vi "Workspace.Initialize.vi"(11 "State":T1) -> (0 "error out":errorcluster, 3 "State":T1)   [LabVIEW 2015, in "J1939 Workspace Object.lvlib"]
uses:
  J1939 Workspace Object.lvlib
  Control Addon/Source/Workspace Objects/Types/UI.StateVariables.ctl
  <vilib>/NI Veristand/Display Template Support/Display Template Support.llb/enum_Display Template Handler Minimal To Widget Msg.ctl
  <vilib>/NI Veristand/Execution/Workspace/SystemStateRegEventRef.ctl
  <vilib>/NI Veristand/Execution/Workspace/Target State Info.ctl
  <vilib>/NI Veristand/Execution/Workspace/Target State.ctl
  Shared/Types/Private Data.ctl
  <vilib>/NI/STM/TCP/TCP Connection Info.ctl
  <vilib>/NI/STM/SubVIs/MetaDataElement.ctl
  Shared/Types/Error Cluster.ctl
  Shared/Types/Error Types.ctl
  NationalInstruments.VeriStand.SystemStorage
  <vilib>/NI Veristand/Display Template Support/Display Template Support.llb/enum_Display Template Handler Minimal To Workspace.ctl
  <vilib>/NI Veristand/Execution/Workspace/WorkspaceAPI.ctl
  NationalInstruments.VeriStand.ClientAPI
  <vilib>/NI Veristand/Execution/Workspace/SystemStateEventRef.ctl
  Control Addon/Source/Workspace Objects/Types/UI.Refs.ctl
  <vilib>/NI Veristand/Execution/Workspace/NI_VS Workspace ExecutionAPI.lvlib
  Shared/J1939 Addon Shared.lvlib
  <vilib>/NI/STM/NI STM.lvlib
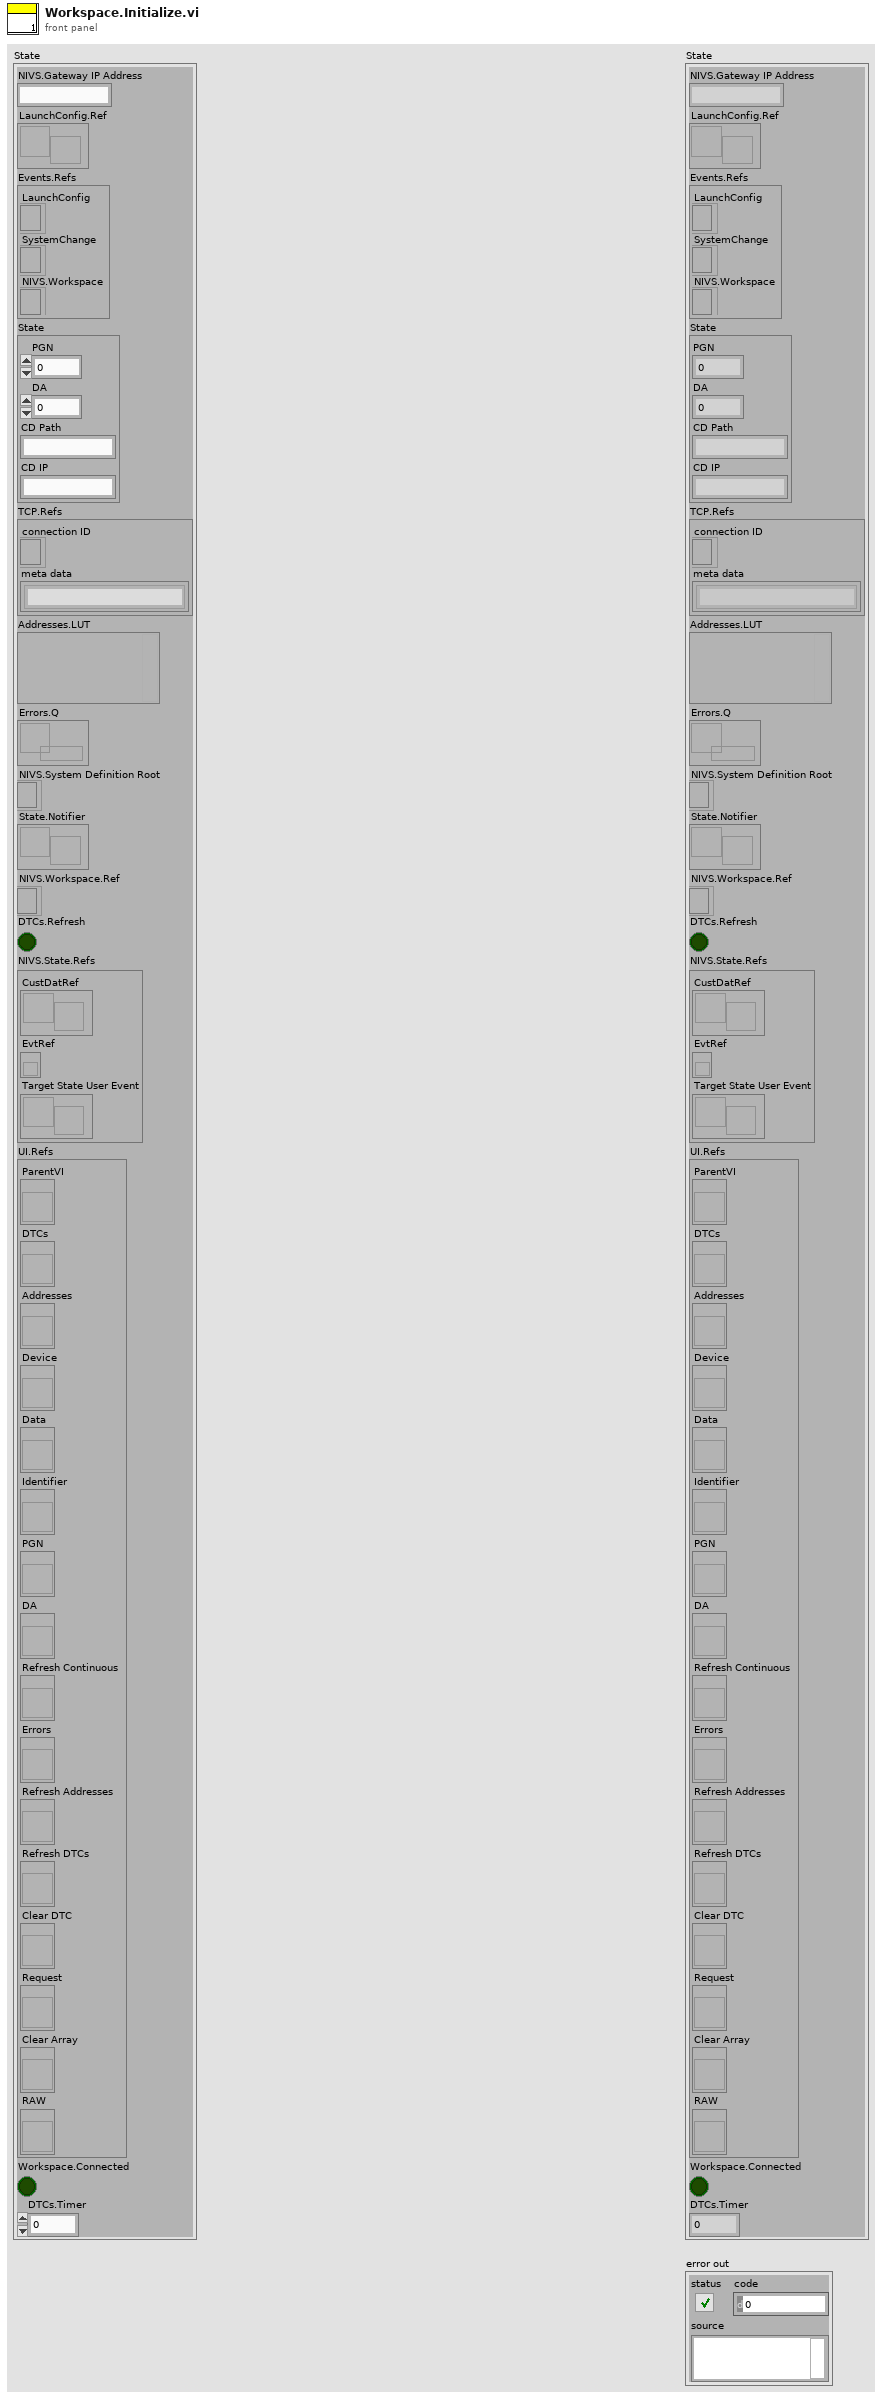
[diagram p1: front panel]
types:
  T1 = typedef "J1939 Workspace Object.lvlib/UI.StateVariables.ctl" = cluster{"NIVS.Gateway IP Address":string, "LaunchConfig.Ref":refnum<user-event>, "Events.Refs":cluster{"LaunchConfig":refnum<event-registration>, "SystemChange":T2, "NIVS.Workspace":refnum<event-registration>}, "State":T3, "TCP.Refs":T4, "Addresses.LUT":variant, "Errors.Q":refnum<queue>, "NIVS.System Definition Root":refnum<k24>, "State.Notifier":refnum<user-event>, "NIVS.Workspace.Ref":T6, "DTCs.Refresh":bool, "NIVS.State.Refs":T7, "UI.Refs":T8, "Workspace.Connected":bool, "DTCs.Timer":u32}
  T2 = typedef "NI_VS Workspace ExecutionAPI.lvlib/SystemStateRegEventRef.ctl" = refnum<event-registration>
  T3 = typedef "J1939 Addon Shared.lvlib/Private Data.ctl" = cluster{"PGN":u32, "DA":u8, "CD Path":string, "CD IP":string}
  T4 = typedef "NI STM.lvlib/TCP Connection Info.ctl" = cluster{"connection ID":refnum<k5>, "meta data":T5[]}
  T5 = typedef "NI STM.lvlib/MetaDataElement.ctl" = string
  T6 = typedef "NI_VS Workspace ExecutionAPI.lvlib/WorkspaceAPI.ctl" = refnum<k24>
  T7 = typedef "NI_VS Workspace ExecutionAPI.lvlib/SystemStateEventRef.ctl" = cluster{"CustDatRef":refnum<user-event>, "EvtRef":refnum<k27>, "Target State User Event":refnum<user-event>}
  T8 = typedef "J1939 Workspace Object.lvlib/UI.Refs.ctl" = cluster{"ParentVI":refnum<vi>, "DTCs":refnum<vi>, "Addresses":refnum<vi>, "Device":refnum<vi>, "Data":refnum<vi>, "Identifier":refnum<vi>, "PGN":refnum<vi>, "DA":refnum<vi>, "Refresh Continuous":refnum<vi>, "Errors":refnum<vi>, "Refresh Addresses":refnum<vi>, "Refresh DTCs":refnum<vi>, "Clear DTC":refnum<vi>, "Request":refnum<vi>, "Clear Array":refnum<vi>, "RAW":refnum<vi>}
  T9 = typedef "J1939 Addon Shared.lvlib/Error Cluster.ctl" = cluster{"error out":errorcluster, "Enum":T10, "Address":u8, "Timestamp":timestamp}
  T10 = typedef "J1939 Addon Shared.lvlib/Error Types.ctl" = enum16{"Request", "RAW Generation", "Clear Active DTCs", "Clear Previous DTCs", "Addresses", "TLAs", "Get Active DTCs", "Get Previous DTCs", "TCP Connection"}
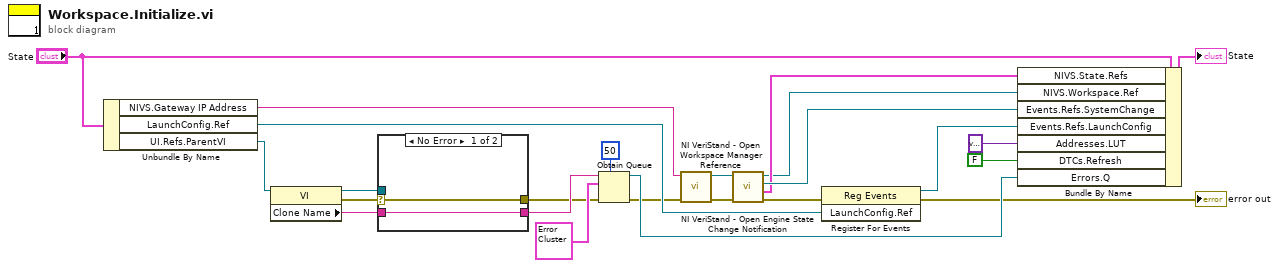
[diagram p0: block diagram]
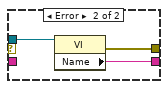
[diagram p2: hidden frame]
diagram:
  n1 = Unbundle By Name("State") -> ("NIVS.Gateway IP Address"=w11:string, "LaunchConfig.Ref"=w22:refnum<user-event>, "UI.Refs.ParentVI"=w7:refnum<vi>)
  n2 = property class="VI"(reference=w7) -> (reference out=w4:refnum<vi>, error out=w5:errorcluster, "Clone Name"=w1:string)  [unwired: 1 in]
  n3 = case shown="No Error" w5 {
    selector: w5 -> [w25 _]
    tunnel: w4 -> [_ w29]
    tunnel: [w26 w28] -> w3
    tunnel: [w25 w27] -> w2
    tunnel: w1 -> [w26 _]
    frame No Error {
    }
    frame Error {
      n4 = property class="VI"(reference=w29) -> (error out=w27:errorcluster, "Name"=w28:string)  [unwired: 1 in, 1 out]
    }
  }
  n5 = Obtain Queue(max queue size (-1, unlimited)=50, name (unnamed)=w3, element data type=T9 {"error out"={"status"=FALSE, "code"=0, "source"=""}, "Enum"=enum."Request", "Address"=0, "Timestamp"=timestamp(0 s since 1904-01-01)} ("Error Cluster"), error in (no error)=w2) -> (queue out=w24:refnum<queue>, error out=w6:errorcluster)  [unwired: 1 in, 1 out]
  n6 = call <vilib>:"NI VeriStand - Open Workspace Manager Reference.vi"("error in (no error)"=w6, "Gateway IP Address (\"\": localhost)"=w11) -> ("error out"=w9:errorcluster, "WorkspaceManager"=w8:T6)  [unwired: 8 in]
  n7 = call <vilib>:"NI VeriStand - Open Engine State Change Notification.vi"("error in (no error)"=w9, "WorkspaceManager in"=w8) -> ("error out"=w10:errorcluster, "SystemStateRefs"=w19:T7, "SystemChangeEventRef"=w21:T2, "WorkspaceManager out"=w13:T6)  [unwired: 6 in]
  n8 = register-events(error in=w10, w22) -> (reference out=w20:refnum<event-registration>, error out=→"error out":errorcluster)  [unwired: 1 in]
  n9 = Bundle By Name(cluster="State", "NIVS.State.Refs"=w19, "NIVS.Workspace.Ref"=w13, "Events.Refs.SystemChange"=w21, "Events.Refs.LaunchConfig"=w20, "Addresses.LUT"=variant ("Addresses"), "DTCs.Refresh"=FALSE, "Errors.Q"=w24) -> (→"State":T1)
